vi "ex_6.vi"() -> ()   [LabVIEW 2020]
panel:
  out "Even elements":i32[](array[numeric])
  out "Odd elements":i32[](array[numeric])
  out "All elements":i32[](array[numeric])
  in  "M":i32
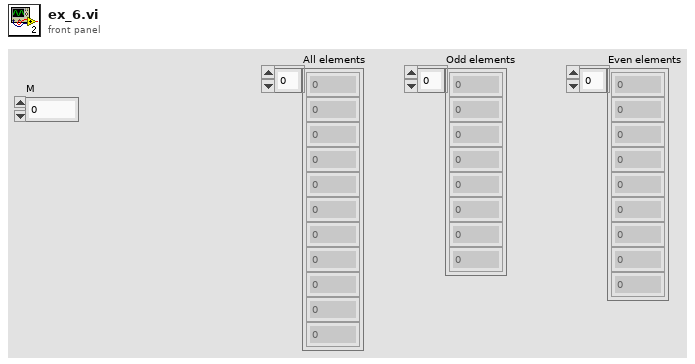
[diagram p1: front panel]
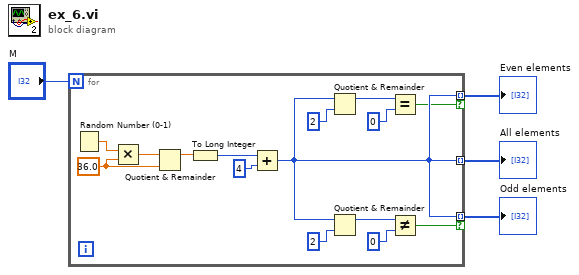
[diagram p0: block diagram]
diagram:
  n1 = for {
    N: "M" -> [_]
    tunnel: [w6] -> w1 mode=indexing if=w12
    tunnel: [w6] -> w3 mode=indexing
    tunnel: [w6] -> w2 mode=indexing if=w5
    w17 = 36.0 ("y")
    n2 = Random Number (0-1)() -> (number: 0 to 1=w19:dbl)
    n3 = Multiply(x=w19, y=w17) -> (x*y=w18:dbl)
    n4 = Quotient & Remainder(x=w18, y=w17) -> (x-y*floor(x/y)=w16:dbl)  [unwired: 1 out]
    n5 = To Long Integer(number=w16) -> (32bit integer=w11:i32)
    n6 = Add(x=w11, y=4) -> (x+y=w6:i32)
    n7 = Quotient & Remainder(x=w6, y=2) -> (x-y*floor(x/y)=w8:i32)  [unwired: 1 out]
    n8 = Quotient & Remainder(x=w6, y=2) -> (x-y*floor(x/y)=w14:i32)  [unwired: 1 out]
    n9 = Equal?(x=w8, y=0) -> (x = y?=w5:bool)
    n10 = Not Equal?(x=w14, y=0) -> (x != y?=w12:bool)
  }
  "All elements" <- w3
  "Odd elements" <- w1
  "Even elements" <- w2
